vi "Convert LV Numeric Representation into DB Type.vi"(10 "Representation":T1) -> (2 "String Value":string)   [LabVIEW 2018, in "ORM Scripter.lvclass"]
uses:
  ORM Scripter.lvclass
  <vilib>/numeric/LVNumericRepresentation.ctl
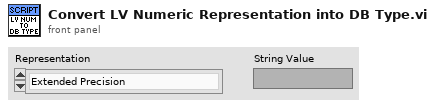
[diagram p1: front panel]
types:
  T1 = typedef "LVNumericRepresentation.ctl" = enum32{"Extended Precision", "Double Precision", "Single Precision", "Long", "Word", "Byte", "Unsigned Long", "Unsigned Word", "Unsigned Byte", "Complex Extended", "Complex Double", "Complex Single", "Quad", "Unsigned Quad", "Fixed-Point"}
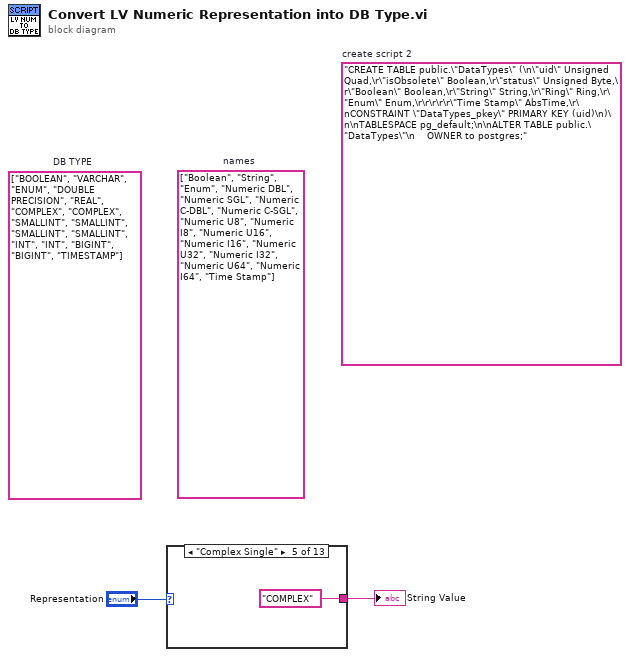
[diagram p0: block diagram]
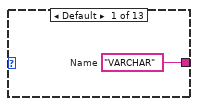
[diagram p2: hidden frame]
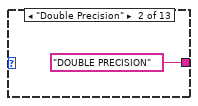
[diagram p3: hidden frame]
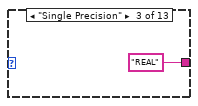
[diagram p4: hidden frame]
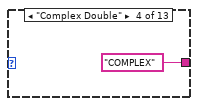
[diagram p5: hidden frame]
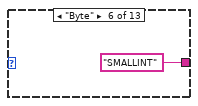
[diagram p6: hidden frame]
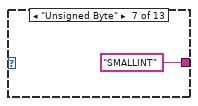
[diagram p7: hidden frame]
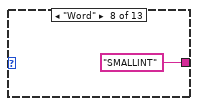
[diagram p8: hidden frame]
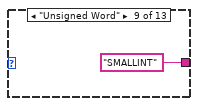
[diagram p9: hidden frame]
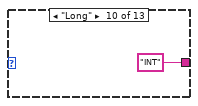
[diagram p10: hidden frame]
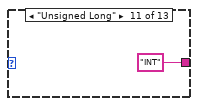
[diagram p11: hidden frame]
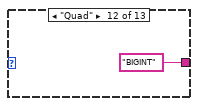
[diagram p12: hidden frame]
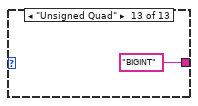
[diagram p13: hidden frame]
diagram:
  (unwired) "CREATE TABLE public.\"DataTypes\" (\n\"uid\" Unsigned Quad,\r\"isObsolete\" Boolean,\r\"status\" Unsigned Byte,\r\"Boolean\" Boolean,\r\"String\" String,\r\"Ring\" Ring,\r\"Enum\" Enum,\r\r\r\r\r\"Time Stamp\" AbsTime,\r\nCONSTRAINT \"DataTypes_pkey\" PRIMARY KEY (uid)\n)\n\nTABLESPACE pg_default;\n\nALTER TABLE public.\"DataTypes\"\n    OWNER to postgres;"  # create script 2
  (unwired) string[] ["Boolean", "String", "Enum", "Numeric DBL", "Numeric SGL", "Numeric C-DBL", "Numeric C-SGL", "Numeric U8", "Numeric I8", "Numeric U16", "Numeric I16", "Numeric U32", "Numeric I32", "Numeric U64", "Numeric I64", "Time Stamp"]  # names
  (unwired) string[] ["BOOLEAN", "VARCHAR", "ENUM", "DOUBLE PRECISION", "REAL", "COMPLEX", "COMPLEX", "SMALLINT", "SMALLINT", "SMALLINT", "SMALLINT", "INT", "INT", "BIGINT", "BIGINT", "TIMESTAMP"]  # DB TYPE
  n1 = case shown="\"Complex Single\"" "Representation" {
    tunnel: [w3 "DOUBLE PRECISION" "REAL" "COMPLEX" "COMPLEX" "SMALLINT" "SMALLINT" "SMALLINT" "SMALLINT" "INT" "INT" "BIGINT" "BIGINT"] -> w1
    frame Default {
      w3 = "VARCHAR"  # Name
    }
    frame "Double Precision" {
    }
    frame "Single Precision" {
    }
    frame "Complex Double" {
    }
    frame "Complex Single" {
    }
    frame "Byte" {
    }
    frame "Unsigned Byte" {
    }
    frame "Word" {
    }
    frame "Unsigned Word" {
    }
    frame "Long" {
    }
    frame "Unsigned Long" {
    }
    frame "Quad" {
    }
    frame "Unsigned Quad" {
    }
  }
  "String Value" <- w1
